vi "Delete Settings.vi"(3 "Scan settings":u16(ring) items=["Regular", "Inverted"], 4 "JV curve scan settings":T1(array[cluster]), 5 "Strings In":string[](array[string])) -> (0 "Scan settings Out":u16(ring) items=["Regular", "Inverted"], 1 "JV curve scan settings Out":T1(array[cluster]), 2 "Strings Out":string[](array[string]))   [LabVIEW 2011]
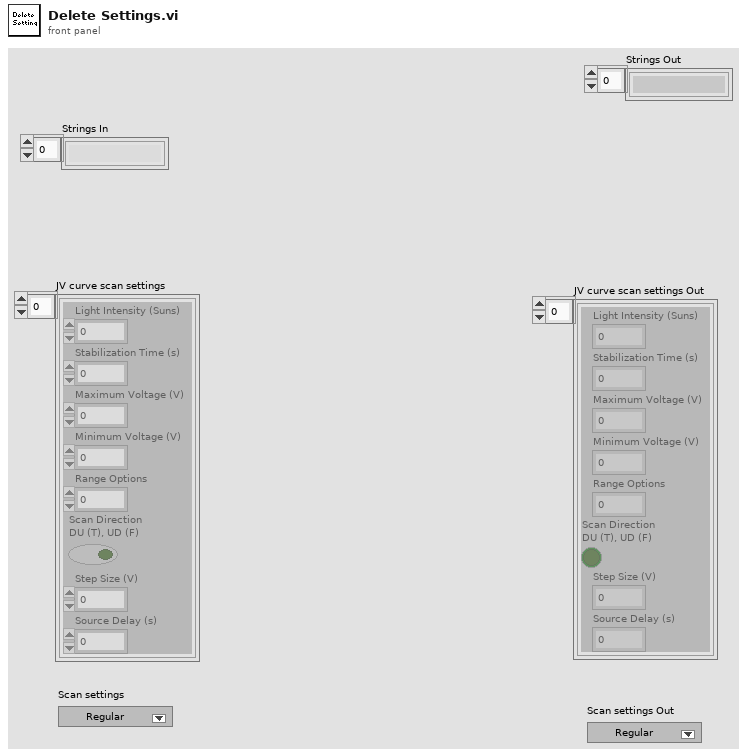
[diagram p1: front panel]
types:
  T1 = cluster{"Light Intensity (Suns)":dbl, "Stabilization Time (s)":dbl, "Maximum Voltage (V)":dbl, "Minimum Voltage (V)":dbl, "Range Options":u16, "Scan Direction\nDU (T), UD (F)":bool, "Step Size (V)":dbl, "Source Delay (s)":dbl}[]
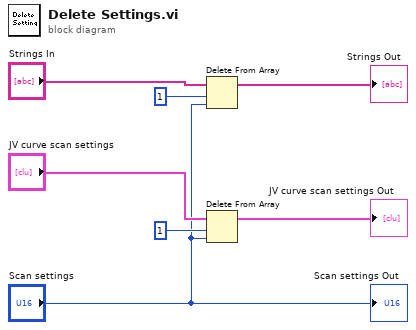
[diagram p0: block diagram]
diagram:
  n1 = Delete From Array(array="Strings In", length=1, index="Scan settings") -> (array with subset deleted=→"Strings Out":string[])  [unwired: 1 out]
  n2 = Delete From Array(array="JV curve scan settings", length=1, index="Scan settings") -> (array with subset deleted=→"JV curve scan settings Out":T1)  [unwired: 1 out]
  "Scan settings Out" <- "Scan settings"
